vi "Null Broadcast Events--constant.vi"() -> (3 "UI Manager Broadcast Events":T1)   [LabVIEW 2020, in "UI Manager.lvlib"]
doc: "Returns the broadcast events cluster with null references for defining the event types in a Register For Events function.\n____\nHAMPEL SOFTWARE ENGINEERING v2.6.0 (2023-12-19 10:54)"
uses:
  UI Manager.lvlib
  Broadcast Events--cluster.ctl
  Did Init Argument--cluster.ctl
  Status Updated Argument--cluster.ctl
  Error Reported Argument--cluster.ctl
  Stop Argument--cluster.ctl
  Get Module Execution Status Argument--cluster.ctl
  System Message Argument--cluster.ctl
  Libraries/hse-libraries/Source/hse-dqmh/Controls/System Message Source.ctl
  Login Argument--cluster.ctl
  Key down Argument--cluster.ctl
  <vilib>/event_ctls.llb/eventvkey.ctl
  Libraries/hse-libraries/Source/hse-dqmh/hse-dqmh.lvlib
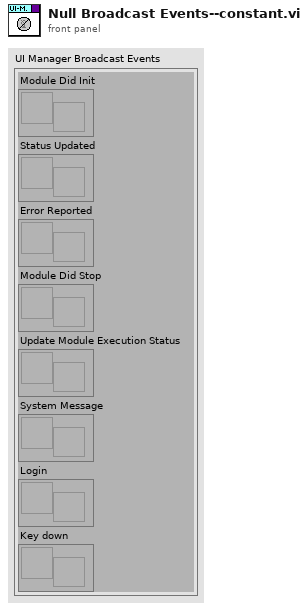
[diagram p1: front panel]
types:
  T1 = typedef "UI Manager.lvlib/Broadcast Events--cluster.ctl" = cluster{"Module Did Init":refnum<user-event>, "Status Updated":refnum<user-event>, "Error Reported":refnum<user-event>, "Module Did Stop":refnum<user-event>, "Update Module Execution Status":refnum<user-event>, "System Message":refnum<user-event>, "Login":refnum<user-event>, "Key down":refnum<user-event>}
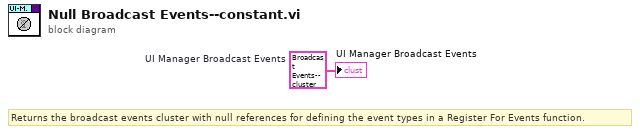
[diagram p0: block diagram]
diagram:
  w1 = T1 {"Module Did Init"=refnum, "Status Updated"=refnum, "Error Reported"=refnum, "Module Did Stop"=refnum, "Update Module Execution Status"=refnum, "System Message"=refnum, "Login"=refnum, "Key down"=refnum}  # UI Manager Broadcast Events
  # "Returns the broadcast events cluster with null references for defining the event types in a Register For Events function."
  "UI Manager Broadcast Events" <- w1
